vi "Register+bit string to range.vi"(10 "Register [MSB:LSB]":string) -> (0 "MIN value":u8, 3 "MAX value":u8, 4 "register":u8 caption="Register" format="0x%x", 5 "LSB":u8, 7 "MSB":u8)   [LabVIEW 2021]
panel:
  out "Bits":string="0x00"
  out "Register":string="0x00"
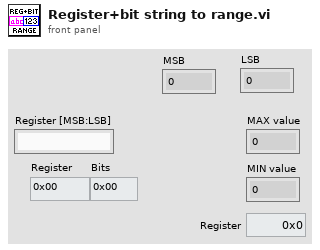
[diagram p1: front panel]
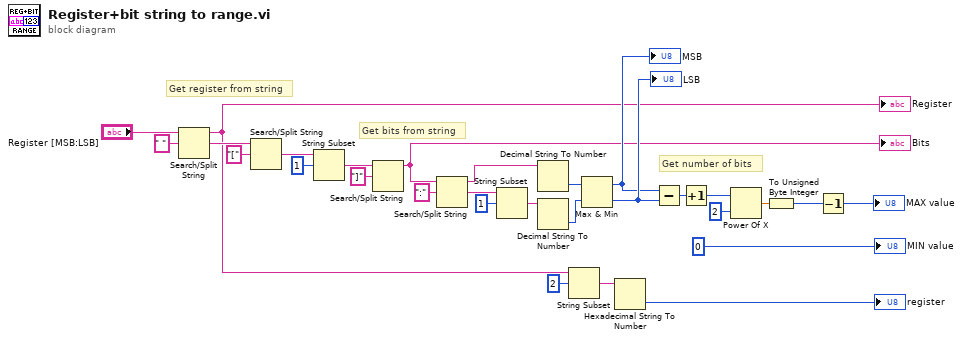
[diagram p0: block diagram]
diagram:
  # "Get number of bits"
  # "Get bits from string"
  # "Get register from string"
  n1 = Search/Split String(string="Register [MSB:LSB]", search string/char (-)=" ") -> (substring before match=w4:string, match + rest of string=w13:string)  [unwired: 1 in, 1 out]
  "Register" <- w4
  n2 = Search/Split String(string=w13, search string/char (-)="[") -> (match + rest of string=w11:string)  [unwired: 1 in, 2 out]
  n3 = String Subset(string=w11, offset (0)=1 ("length (rest)")) -> (substring=w12:string)  [unwired: 1 in]
  n4 = Search/Split String(string=w12, search string/char (-)="]") -> (substring before match=w16:string)  [unwired: 1 in, 2 out]
  "Bits" <- w16
  n5 = Search/Split String(string=w16, search string/char (-)=":") -> (substring before match=w29:string, match + rest of string=w18:string)  [unwired: 1 in, 1 out]
  n6 = String Subset(string=w18, offset (0)=1) -> (substring=w19:string)  [unwired: 1 in]
  n7 = Decimal String To Number(string=w29) -> (number=w20:i32)  [unwired: 2 in, 1 out]
  n8 = Decimal String To Number(string=w19) -> (number=w21:i32)  [unwired: 2 in, 1 out]
  n9 = String Subset(string=w4, offset (0)=2) -> (substring=w5:string)  [unwired: 1 in]
  n10 = Max & Min(x=w20, y=w21) -> (max(x,y)=w22:i32, min(x,y)=w23:i32)
  "MSB" <- w22
  "LSB" <- w23
  n11 = Hexadecimal String To Number(string=w5) -> (number=→"register":u32)  [unwired: 2 in, 1 out]
  n12 = Subtract(x=w22, y=w23) -> (x-y=w24:i32)
  n13 = Increment(x=w24) -> (x+1=w26:i32)
  n14 = Power Of X(1:2 ("x"), 2:w26) -> (0:w28:dbl)
  n15 = To Unsigned Byte Integer(number=w28) -> (unsigned 8bit integer=w2:u8)
  n16 = Decrement(x=w2) -> (x-1=→"MAX value":u8)
  "MIN value" <- u8 0 ("min value")
